vi "dg535 example.vi"(0 "GPIB address":string="15", 1 "A":dbl min=0.0 max=999.999999999995 format="%.12f", 2 "C":dbl min=0.0 max=999.999999999995 format="%.12f", 3 "set":bool, 4 "read and set output":T1={"mode"=0, "load"=FALSE, "inversion"=FALSE, "amplitude"=1.0, "offset"=0.0} {"offset" min=-3.0 max=4.0 format="%.2f"; "amplitude" min=-3.0 max=4.0 format="%.2f"; "mode" items=["TTL", "NIM", "ECL", "VAR"]}, 5 "trigger":T2={"trigger"=0, "internal/burst trigger rate"=0.001, "burst period"=4, "external trigger level"=0.0, "burst count"=2, "trigger slope"=FALSE, "input impedance"=FALSE} {"trigger" scale=0.0..4.0; "burst count" min=2 max=32766; "external trigger level" min=-2.56 max=2.56 format="%.2f"; "burst period" min=4 max=32766; "internal/burst trigger rate" min=0.001 max=1000000.0 format="%.3f"}, 7 "delay":cluster{"A=":u32, "B=":u32, "C=":u32, "D=":u32} {"D=" scale=0.0..3.0; "C=" scale=0.0..3.0; "A=" scale=0.0..3.0; "B=" scale=0.0..3.0}, 9 "output":u16(ring) items=["T0", "A", "B", "AB", "C", "D", "CD"], 11 "error in":errorcluster, 12 "B":dbl min=0.0 max=999.999999999995 format="%.12f", 13 "D":dbl min=0.0 max=999.999999999995 format="%.12f", 14 "read":bool) -> (15 "error out":errorcluster)   [LabVIEW 2011]
doc: "This VI is an example of how to use the DG535 subVIs programmatically .\nThe DG535 TRIGGER.VI sets the trigger mode , internal/burst trigger rate , burst count , burst period , external threshold voltage , external trigger slope and impedance of the DG535 .\nErrors are reported if the trigger rate is too high or if the burst period is out-of-range .\nThe DG535 DELAY.VI sets the delay time of channel i to t seconds relative to channel j . A \"Delay Linkage Error\" is caused by an attempt to totally disconnect a time reference from T0 . A \"Delay Range Error\" is reported when the total time delay for a channel exceeds 999.999999999995 seconds .\nDG535 SET OUTPUT.VI sets the mode , load , output polarity, amplitude and offset of the OUTPUT BNC selected while the DG535 READ OUTPUT.VI reads and displays these values ."
panel:
  # "DG535 FOUR CHANNEL DIGITAL DELAY/PULSE GENERATOR"
  # "50 Ohm\nHigh Z"
  # "50 Ohm\nHigh Z"
  # "-ve edge\n+ve  edge"
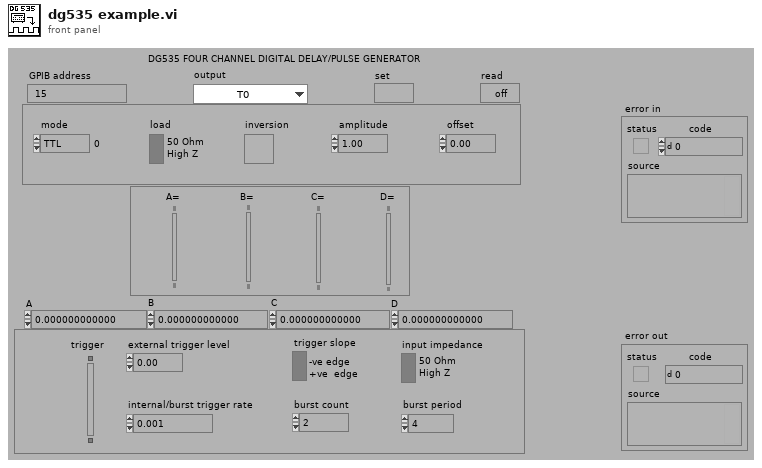
[diagram p1: front panel]
types:
  T1 = cluster{"mode":i32, "load":bool, "inversion":bool, "amplitude":dbl, "offset":dbl}
  T2 = cluster{"trigger":u32, "internal/burst trigger rate":dbl, "burst period":i32, "external trigger level":sgl, "burst count":i32, "trigger slope":bool, "input impedance":bool}
  T3 = cluster{"mode":u8, "load":bool, "inversion":bool, "amplitude":dbl, "offset":dbl}
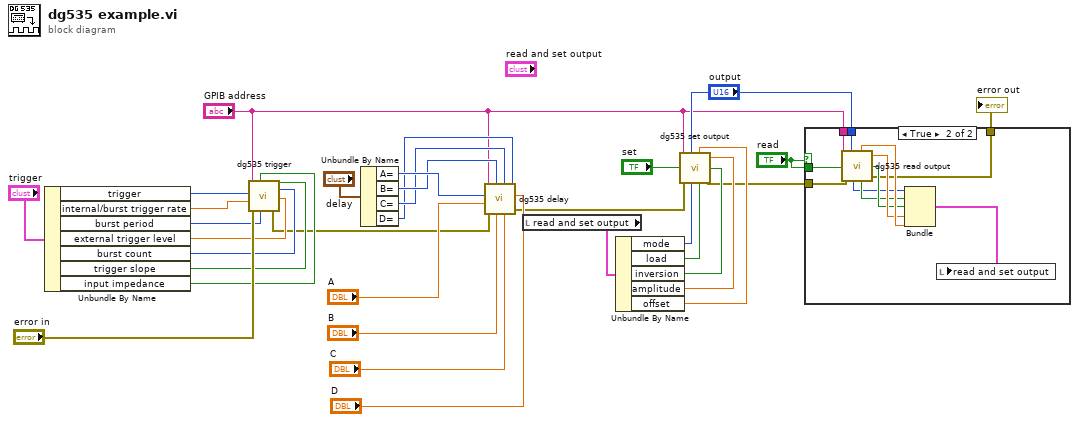
[diagram p0: block diagram]
diagram:
  n1 = Unbundle By Name("trigger") -> ("trigger"=w31:u32, "internal/burst trigger rate"=w30:dbl, "burst period"=w28:i32, "external trigger level"=w27:sgl, "burst count"=w26:i32, "trigger slope"=w25:bool, "input impedance"=w24:bool)
  n2 = call "dg535 trigger.vi"("external trigger level"=w27, "burst count"=w26, "trigger slope"=w25, "burst period"=w28, "input impedance"=w24, "error in"="error in", "internal/burst trigger rate"=w30, "trigger"=w31, "GPIB address"="GPIB address") -> ("error out"=w20:errorcluster)
  n3 = Unbundle By Name("delay") -> ("A="=w22:u32, "B="=w19:u32, "C="=w17:u32, "D="=w14:u32)
  n4 = call "dg535 delay.vi"("C"="C", "D"="D", "D="=w14, "C="=w17, "B"="B", "error in"=w20, "A"="A", "B="=w19, "A="=w22, "GPIB address"="GPIB address") -> ("error out"=w6:errorcluster)
  n5 = local read "read and set output"() -> (w8:T1)
  n6 = Unbundle By Name(w8) -> ("mode"=w13:i32, "load"=w12:bool, "inversion"=w11:bool, "amplitude"=w10:dbl, "offset"=w9:dbl)
  n7 = call "dg535 set output.vi"("GPIB address"="GPIB address", "output"="output", "set"="set", "error in"=w6, "mode"=w13, "offset"=w9, "amplitude"=w10, "inversion"=w11, "load"=w12) -> ("error out"=w5:errorcluster)
  n8 = case shown="True" "read" {
    tunnel: w5 -> [w33 w39]
    tunnel: [w33 w38] -> w4
    tunnel: "read" -> [_ w37]
    tunnel: "output" -> [_ w36]
    tunnel: "GPIB address" -> [_ w35]
    frame False {
    }
    frame True {
      n9 = call "dg535 read output.vi"("GPIB address"=w35, "output"=w36, "read"=w37, "error in"=w39) -> ("mode"=w34:u8, "offset"=w43:dbl, "amplitude"=w42:dbl, "inversion"=w41:bool, "load"=w40:bool, "error out"=w38:errorcluster)
      n10 = Bundle("mode"=w34, "load"=w40, "inversion"=w41, "amplitude"=w42, "offset"=w43) -> (w44:T3)  [unwired: 1 in]
      n11 = local write "read and set output"(w44) -> ()
    }
  }
  "error out" <- w4
